vi "obtener_Telemetria.vi"(7 "Enc_values_in":T1, 8 "error in":errorcluster, 10 "Cluster_modbus":T5, 11 "new_data?":bool) -> (0 "error out":errorcluster, 5 "Enc_values_out":T1)   [LabVIEW 2026]
uses:
  Control/Ctrl_Modbus28.ctl
  Control/Ctr_Enc_Values.ctl
  Control/Ctrl_datos6motores_final.ctl
  Control/Ctrl_Motores_Valores.ctl
  Control/Ctrl_Errores.ctl
  <vilib>/ptbypt/NI_PtbyPt.lvlib
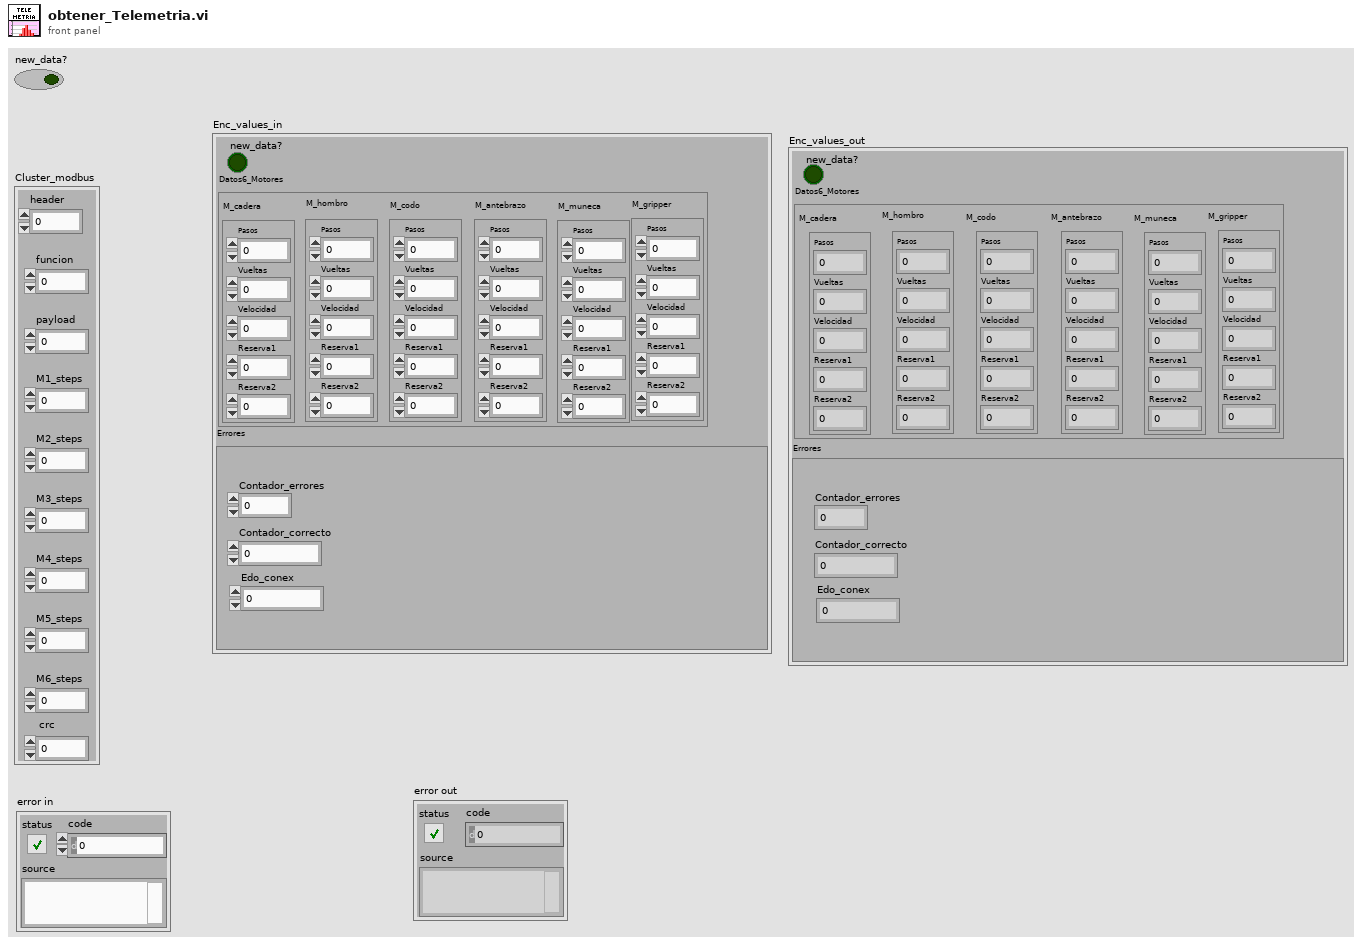
[diagram p1: front panel]
types:
  T1 = typedef "Ctr_Enc_Values.ctl" = cluster{"Datos6_Motores":T2, "Errores":T4, "new_data?":bool}
  T2 = typedef "Ctrl_datos6motores_final.ctl" = cluster{"M_cadera":T3, "M_hombro":T3, "M_codo":T3, "M_antebrazo":T3, "M_muneca":T3, "M_gripper":T3}
  T3 = typedef "Ctrl_Motores_Valores.ctl" = cluster{"Pasos":i32, "Vueltas":i16, "Velocidad":dbl, "Reserva1":u8, "Reserva2":u8}
  T4 = typedef "Ctrl_Errores.ctl" = cluster{"Contador_correcto":u32, "Contador_errores":u32, "Edo_conex":u32}
  T5 = typedef "Ctrl_Modbus28.ctl" = cluster{"header":u8, "funcion":u8, "payload":u8, "M1_steps":i32, "M2_steps":i32, "M3_steps":i32, "M4_steps":i32, "M5_steps":i32, "M6_steps":i32, " crc":u8}
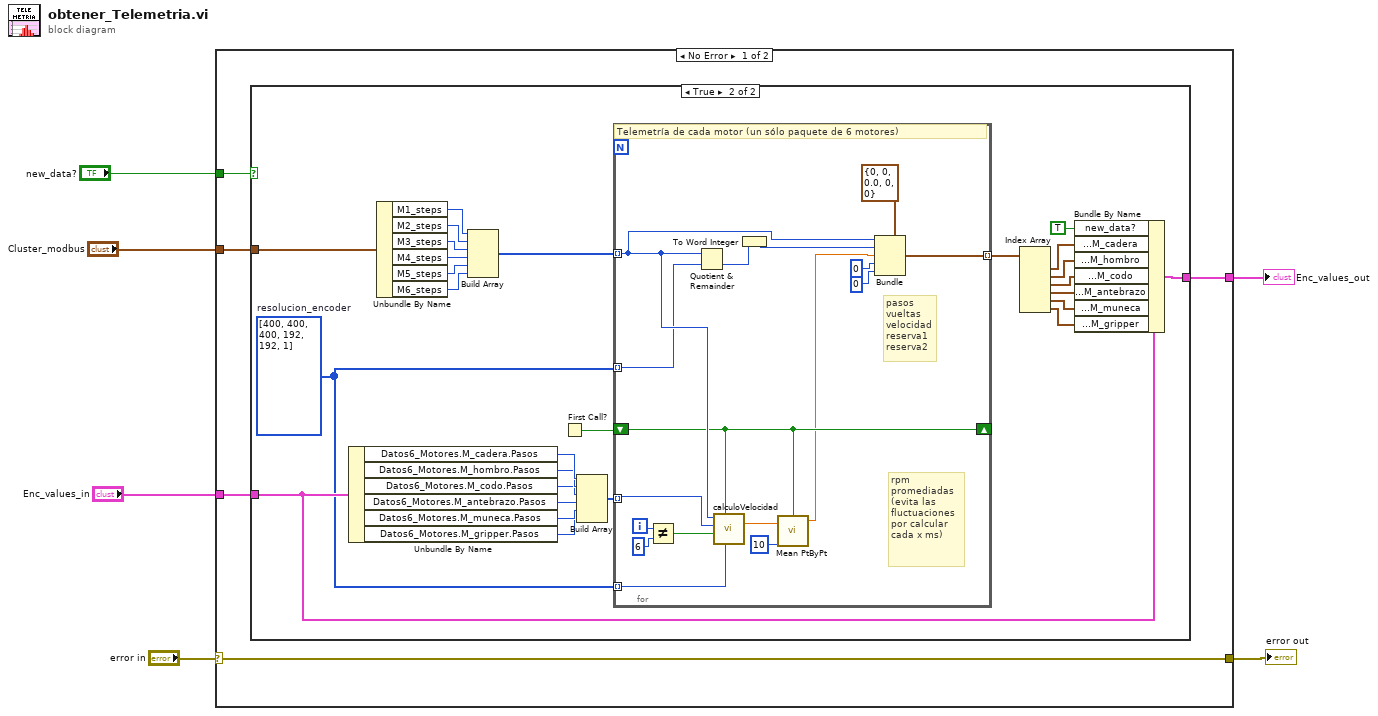
[diagram p0: block diagram]
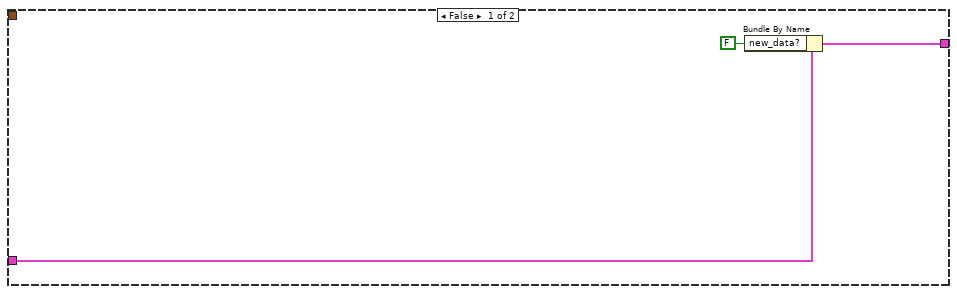
[diagram p2: hidden frame]
diagram:
  n1 = case shown="No Error" "error in" {
    selector: "error in" -> [w11 w60]
    tunnel: [w11 w60] -> w5
    tunnel: "Cluster_modbus" -> [w10 _]
    tunnel: "new_data?" -> [w9 _]
    tunnel: "Enc_values_in" -> [w8 w59]
    tunnel: [w7 w59] -> w1
    frame No Error {
      n2 = case shown="True" w9 {
        tunnel: w10 -> [_ w41]
        tunnel: w8 -> [w13 w25]
        tunnel: [w14 w18] -> w7
        frame False {
          n3 = Bundle By Name(cluster=w13, "new_data?"=FALSE) -> (w14:T1)
        }
        frame True {
          w16 = i32[] [400, 400, 400, 192, 192, 1]  # resolucion_encoder
          n4 = Unbundle By Name(w25) -> ("Datos6_Motores.M_cadera.Pasos"=w33:i32, "Datos6_Motores.M_hombro.Pasos"=w32:i32, "Datos6_Motores.M_codo.Pasos"=w31:i32, "Datos6_Motores.M_antebrazo.Pasos"=w30:i32, "Datos6_Motores.M_muneca.Pasos"=w29:i32, "Datos6_Motores.M_gripper.Pasos"=w28:i32)
          n5 = Unbundle By Name(w41) -> ("M1_steps"=w40:i32, "M2_steps"=w39:i32, "M3_steps"=w38:i32, "M4_steps"=w37:i32, "M5_steps"=w36:i32, "M6_steps"=w35:i32)
          n6 = Build Array(w40, w39, w38, w37, w36, w35) -> (w34:i32[])
          n7 = First Call?() -> (First Call?: T/F=w15:bool)
          n8 = Build Array(w33, w32, w31, w30, w29, w28) -> (w27:i32[])
          n9 = for {
            tunnel: w34 -> [w54] mode=indexing
            tunnel: w16 -> [w50] mode=indexing
            tunnel: w27 -> [w57] mode=indexing
            tunnel: [w56] -> w26 mode=indexing
            tunnel: w16 -> [w49] mode=indexing
            shift-right: [w44] -> _
            shift-left: w15 -> [w44]
            i -> [w48]
            # "rpm promediadas\n(evita las fluctuaciones por calcular cada x ms)"
            # "pasos\nvueltas\nvelocidad\nreserva1\nreserva2"
            # "Telemetría de cada motor (un sólo paquete de 6 motores)"
            n10 = Not Equal?(x=w48, y=6) -> (x != y?=w45:bool)
            n11 = Quotient & Remainder(x=w54, y=w50) -> (floor(x/y)=w58:i32)  [unwired: 1 out]
            n12 = call "calculoVelocidad.vi"("Resolucion"=w49, "primera_iteracion?"=w44, "motor_gripper?"=w45, "Pasos_anteriores"=w57, "Pasos_nuevos"=w54) -> ("RPM"=w43:dbl)  [unwired: 6 in]
            n13 = To Word Integer(number=w58) -> (16bit integer=w53:i16)
            n14 = call <vilib>:"Mean PtByPt.vi"("x"=w43, "sample length"=10, "initialize"=w44) -> ("mean"=w42:dbl)  [unwired: 1 in, 1 out]
            n15 = Bundle(cluster=T3 {"Pasos"=0, "Vueltas"=0, "Velocidad"=0.0, "Reserva1"=0, "Reserva2"=0} ("M_gripper"), "Pasos"=w54, "Vueltas"=w53, "Velocidad"=w42, "Reserva1"=u8 0, "Reserva2"=u8 0) -> (w56:T3)
          }
          n16 = Index Array(array=w26) -> (element #1=w24:T3, element #2=w23:T3, element #3=w22:T3, element #4=w21:T3, element #5=w20:T3, element #6=w19:T3)  [unwired: 6 in]
          n17 = Bundle By Name(cluster=w25, "new_data?"=TRUE, "Datos6_Motores.M_cadera"=w24, "Datos6_Motores.M_hombro"=w23, "Datos6_Motores.M_codo"=w22, "Datos6_Motores.M_antebrazo"=w21, "Datos6_Motores.M_muneca"=w20, "Datos6_Motores.M_gripper"=w19) -> (w18:T1)
        }
      }
    }
    frame Error {
    }
  }
  "error out" <- w5
  "Enc_values_out" <- w1
